vi "NA_save_201216.vi"() -> ()   [LabVIEW 2017]
panel:
  in  "Time Delay":dbl format="%#_13g"
  in  "File Path":string="C:\\NA_Measurements\\Temp\\test.s2p"
  in  "VISA name for M9374A":refnum<visa-resource-name>="TCPIP0::WINDOWS-VQFA9LI::hislip0::INSTR"
  # "M9374A Network Analizer"
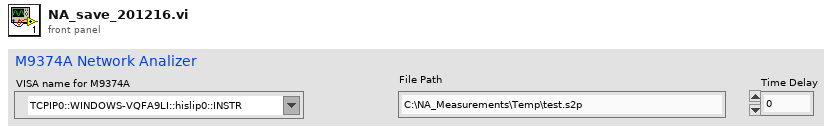
[diagram p1: front panel]
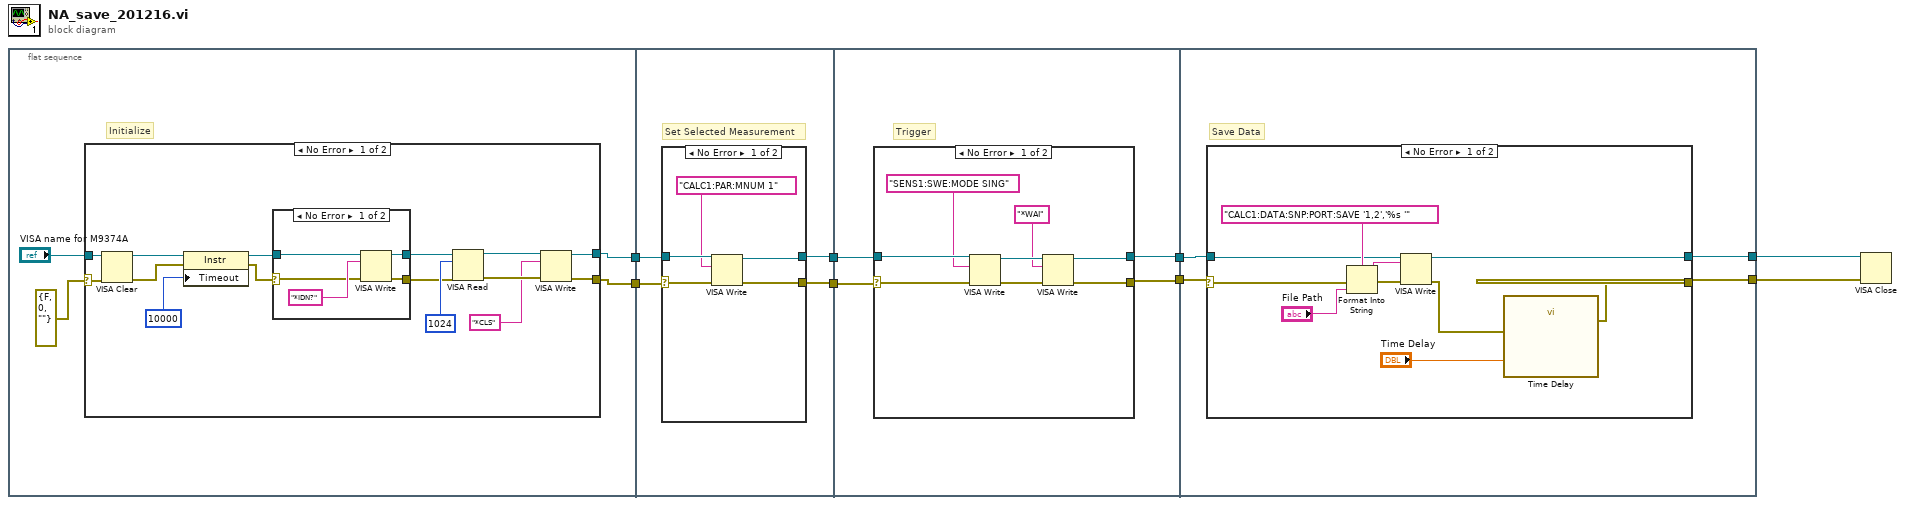
[diagram p0: block diagram]
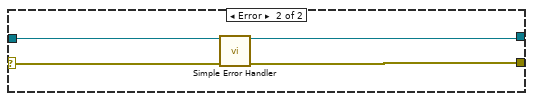
[diagram p3: hidden frame]
diagram:
  n1 = flat-sequence {
    tunnel: [w10] -> w6
    tunnel: [w9] -> w4
    tunnel: w6 -> [w41]
    tunnel: [w39] -> w5
    tunnel: w4 -> [w40]
    tunnel: [w38] -> w3
    tunnel: w5 -> [w52]
    tunnel: w3 -> [w51]
    tunnel: [w50] -> w8
    tunnel: [w49] -> w7
    tunnel: w8 -> [w65]
    tunnel: w7 -> [w66]
    tunnel: [w64] -> w2
    tunnel: [w63] -> w1
    frame #0 {
      # "Initialize"
      n2 = case shown="No Error" errorcluster {"status"=FALSE, "code"=0, "source"=""} ("error in") {
        selector: errorcluster {"status"=FALSE, "code"=0, "source"=""} ("error in") -> [w27 w37]
        tunnel: [w18 w36] -> w9
        tunnel: [w19 w35] -> w10
        tunnel: "VISA name for M9374A" -> [w17 w35]
        frame No Error {
          n3 = VISA Clear(VISA resource name=w17, error in (no error)=w27) -> (VISA resource name out=w26:refnum<visa-resource-name>, error out=w25:errorcluster)
          n4 = property class="Instr"(reference=w26, error in=w25, "Timeout"=u32 10000 ("General Settings:Timeout Value")) -> (reference out=w14:refnum<visa-resource-name>, error out=w13:errorcluster)
          n5 = case shown="No Error" w13 {
            selector: w13 -> [w31 w33]
            tunnel: [w29 w33] -> w15
            tunnel: [w30 w34] -> w16
            tunnel: w14 -> [w28 w34]
            frame No Error {
              n6 = VISA Write(VISA resource name=w28, write buffer="*IDN?" ("Cmds"), error in (no error)=w31) -> (VISA resource name out=w30:refnum<visa-resource-name>, error out=w29:errorcluster)  [unwired: 1 out]
            }
            frame Error {
            }
          }
          n7 = VISA Read(VISA resource name=w16, byte count=1024, error in (no error)=w15) -> (VISA resource name out=w22:refnum<visa-resource-name>, error out=w21:errorcluster)  [unwired: 2 out]
          n8 = VISA Write(VISA resource name=w22, write buffer="*CLS" ("Cmds"), error in (no error)=w21) -> (VISA resource name out=w19:refnum<visa-resource-name>, error out=w18:errorcluster)  [unwired: 1 out]
        }
        frame Error {
          n9 = call <vilib>:"Simple Error Handler.vi"("error in (no error)"=w37) -> ("error out"=w36:errorcluster)  [unwired: 4 in, 4 out]
        }
      }
    }
    frame #1 {
      # "Set Selected Measurement"
      n10 = case shown="No Error" w40 {
        selector: w40 -> [w46 w48]
        tunnel: [w42 w48] -> w38
        tunnel: w41 -> [w45 w47]
        tunnel: [w43 w47] -> w39
        frame No Error {
          n11 = VISA Write(VISA resource name=w45, write buffer="CALC1:PAR:MNUM 1" ("Cmdline"), error in (no error)=w46) -> (VISA resource name out=w43:refnum<visa-resource-name>, error out=w42:errorcluster)  [unwired: 1 out]
        }
        frame Error {
        }
      }
    }
    frame #2 {
      # "Trigger"
      n12 = case shown="No Error" w51 {
        selector: w51 -> [w59 w62]
        tunnel: [w56 w62] -> w49
        tunnel: w52 -> [w60 w61]
        tunnel: [w54 w61] -> w50
        frame No Error {
          n13 = VISA Write(VISA resource name=w60, write buffer="SENS1:SWE:MODE SING" ("Cmdline"), error in (no error)=w59) -> (VISA resource name out=w55:refnum<visa-resource-name>, error out=w57:errorcluster)  [unwired: 1 out]
          n14 = VISA Write(VISA resource name=w55, write buffer="*WAI" ("Cmdline"), error in (no error)=w57) -> (VISA resource name out=w54:refnum<visa-resource-name>, error out=w56:errorcluster)  [unwired: 1 out]
        }
        frame Error {
        }
      }
    }
    frame #3 {
      # "Save Data"
      n15 = case shown="No Error" w66 {
        selector: w66 -> [w72 w78]
        tunnel: [w68 w78] -> w64
        tunnel: w65 -> [w71 w77]
        tunnel: [w70 w77] -> w63
        frame No Error {
          n16 = Format Into String(format string="CALC1:DATA:SNP:PORT:SAVE '1,2','%s '" ("Cmdline"), error in=w72, "File Path") -> (resulting string=w76:string, error out=w75:errorcluster)  [unwired: 1 in]
          n17 = VISA Write(VISA resource name=w71, write buffer=w76, error in (no error)=w75) -> (VISA resource name out=w70:refnum<visa-resource-name>, error out=w69:errorcluster)  [unwired: 1 out]
          n18 = call "Time Delay"("error in (no error)"=w69, "Delay Time (s)"="Time Delay") -> ("error out"=w68:errorcluster)  [unwired: 9 in]
        }
        frame Error {
        }
      }
    }
  }
  n19 = VISA Close(VISA resource name=w1, error in (no error)=w2) -> ()  [unwired: 1 out]
